vi "SENS_IF_FREQ_VAL.vi"(0 "VISA IN":refnum<visa-resource-name>, 1 "Frq. Value":i32, 5 "error in":errorcluster, 7 "Channel":i32) -> (14 "VISA Out":refnum<visa-resource-name>, 19 "error out":errorcluster)   [LabVIEW 2018, in "PNA-X.lvlib"]
doc: "SENSe<cnum>:IF:FREQuency[:VALue] <value> \n(Read-Write) Sets and returns the IF frequency for ALL receiver paths being used for the specified \nchannel. To set this frequency, SENS:IF:FREQ:AUTO must be set to OFF (Manual). \nAlso returns the maximum and minimum allowable frequency settings. \nCritical Note \nParameters \n<cnum> Existing channel number. If unspecified, <cnum> is set to 1. \n<value> (Numeric) Frequency value. \nExamples SENS:IF:FREQ \nsense2:if:frequency \nQuery Syntax SENSe<cnum>:IF:FREQuency? \n'returns the current frequency setting"
uses:
  PNA-X.lvlib
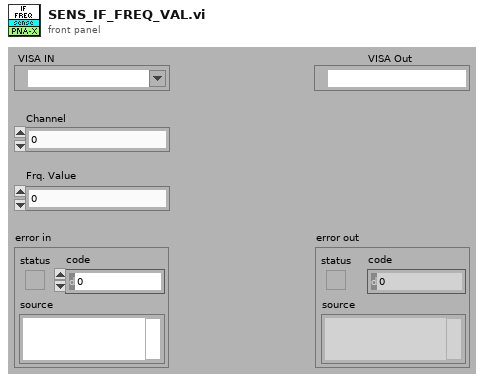
[diagram p1: front panel]
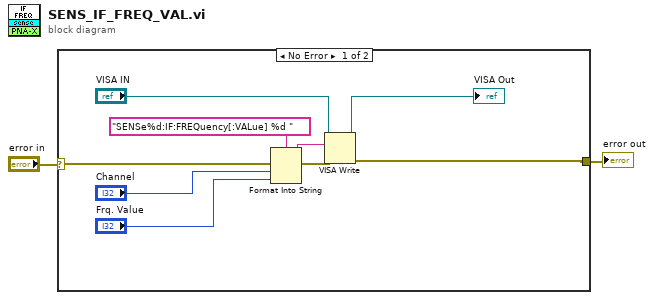
[diagram p0: block diagram]
diagram:
  n1 = case shown="No Error" "error in" {
    selector: "error in" -> [w11 w12]
    tunnel: [w6 w12] -> w1
    frame No Error {
      n2 = Format Into String(format string="SENSe%d:IF:FREQuency[:VALue] %d " ("Cmdline"), error in=w11, "Channel", "Frq. Value") -> (resulting string=w9:string, error out=w10:errorcluster)  [unwired: 1 in]
      n3 = VISA Write(VISA resource name="VISA IN", write buffer=w9, error in (no error)=w10) -> (VISA resource name out=→"VISA Out":refnum<visa-resource-name>, error out=w6:errorcluster)  [unwired: 1 out]
    }
    frame Error {
    }
  }
  "error out" <- w1
